vi "Write Enable.vi"(8 "error in (no error)":errorcluster, 10 "Enable":bool, 11 "CsvReportPlugin in":refnum<class "CsvReportPlugin.lvclass">) -> (0 "error out":errorcluster, 3 "CsvReportPlugin out":refnum<class "CsvReportPlugin.lvclass">)   [LabVIEW 2015, in "CsvReportPlugin.lvclass"]
uses:
  CsvReportPlugin.lvclass
  CsvReportPlugin.lvclass/CsvReportPlugin.ctl
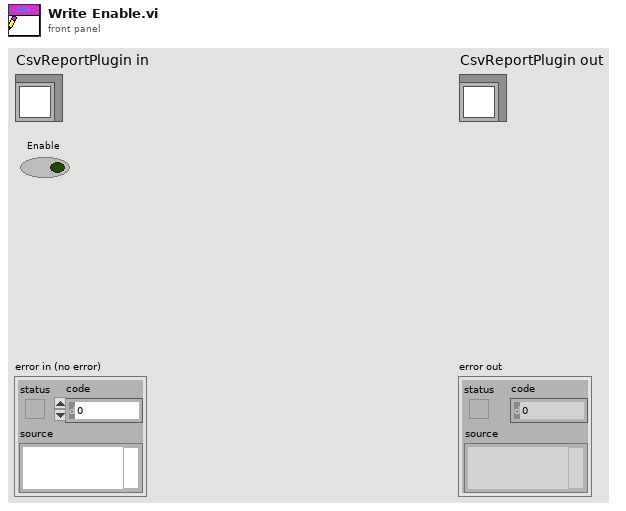
[diagram p1: front panel]
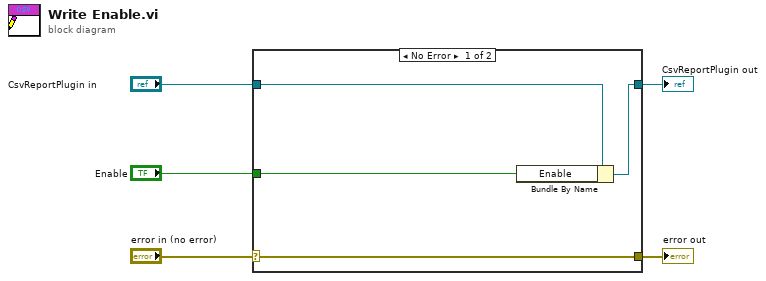
[diagram p0: block diagram]
diagram:
  n1 = case shown="No Error" "error in (no error)" {
    selector: "error in (no error)" -> [w9 w10]
    tunnel: [w9 w10] -> w4
    tunnel: [w7 w11] -> w2
    tunnel: "CsvReportPlugin in" -> [w8 w11]
    tunnel: "Enable" -> [w6 _]
    frame No Error {
      n2 = Bundle By Name(cluster=w8, "Enable"=w6) -> (w7:refnum<class "CsvReportPlugin.lvclass">)
    }
    frame Error {
    }
  }
  "error out" <- w4
  "CsvReportPlugin out" <- w2
